vi "Utility Setup.vi"(8 "error in":errorcluster, 11 "VISA resource name":refnum<visa-resource-name>) -> (0 "error out":errorcluster, 3 "VISA resource name out":refnum<visa-resource-name>)   [LabVIEW 2011, in "GPT-9000.lvlib"]
uses:
  <instrlib>/GPT-9000/GPT-9000.lvlib
panel:
  in  "Setup Buzzer Sound for FAIL":T1={"Buzzer Sound"=0, "Duration Time(Sec)"=0.5} {"Duration Time(Sec)" min=0.2 max=999.9 step=0.1 format="%#.1f"; "Buzzer Sound" format="%b" items=["ON"=1, "OFF"=0]}
  in  "Setup Buzzer Sound for PASS":T1={"Buzzer Sound"=0, "Duration Time(Sec)"=0.5000000029802322} {"Duration Time(Sec)" min=0.20000000298023224 max=999.9000244140625 step=0.1 format="%#.1f"; "Buzzer Sound" format="%b" items=["ON"=1, "OFF"=0]}
  in  "Sets the brightness":u8(ring)=2 items=["bright"=2, "drak"=1]
  in  "Sets the contrast":u8(ring)=8 items=["8"=8, "7"=7, "6"=6, "5"=5, "4"=4, "3"=3, "2"=2, "1"=1]
  in  "SETUP":bool
  out "Query Buzzer Sound for FAIL":T2
  out "Query Buzzer Sound for PASS":T3
  out "Query the brightness":string
  out "Query the contrast":string
  out "ID Return String":string
  in  "Configure RS232 Baud Rate":u32(ring)=9600 items=["9600"=9600, "19200"=19200, "38400"=38400, "57600"=57600, "115200"=115200]
  in  "Clear Error(True)":bool=TRUE
  in  "ID Query (True)":bool=TRUE
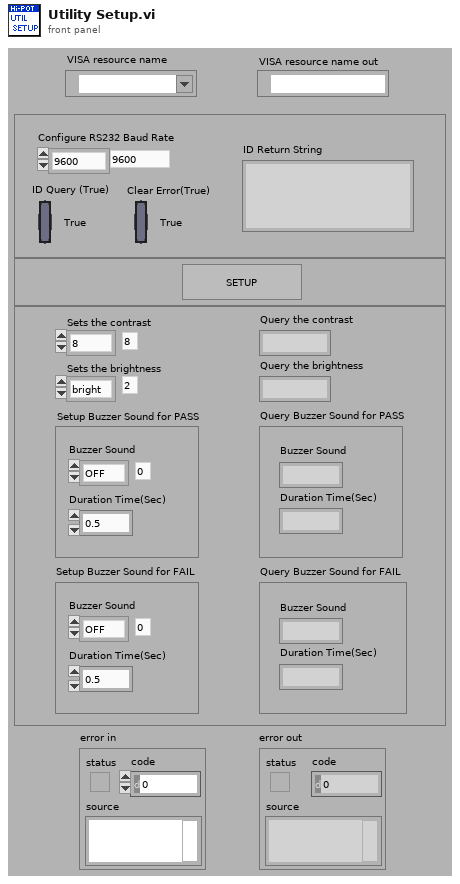
[diagram p1: front panel]
types:
  T1 = cluster{"Buzzer Sound":u8, "Duration Time(Sec)":dbl}
  T2 = cluster{"Duration Time(Sec)":string, "Buzzer Sound":string}
  T3 = cluster{"Buzzer Sound":string, "Duration Time(Sec)":string}
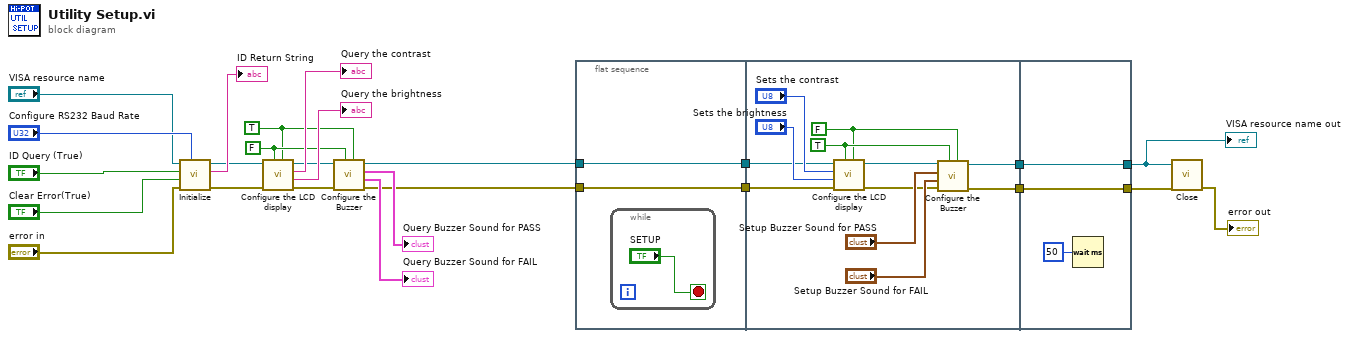
[diagram p0: block diagram]
diagram:
  w6 = TRUE ("Enable to Query")
  w7 = FALSE ("Enable to Setup")
  n1 = call <instrlib>:"Initialize.vi"("Configure RS232 Baud Rate"="Configure RS232 Baud Rate", "error in (no error)"="error in", "Clear Error(True)"="Clear Error(True)", "ID Query (True)"="ID Query (True)", "VISA resource name"="VISA resource name") -> ("error out"=w14:errorcluster, "ID Return String"=→"ID Return String":string, "VISA resource name out"=w15:refnum<visa-resource-name>)  [unwired: 3 in, 1 out]
  n2 = call <instrlib>:"Configure the LCD display.vi"("Enable to Query"=w6, "Enable to Setup"=w7, "error in"=w14, "VISA resource name"=w15) -> ("error out"=w12:errorcluster, "Query the brightness"=→"Query the brightness":string, "Query the contrast"=→"Query the contrast":string, "VISA resource name out"=w13:refnum<visa-resource-name>)  [unwired: 4 in]
  n3 = call <instrlib>:"Configure the Buzzer.vi"("Enable to Query"=w6, "Enable to Setup"=w7, "error in"=w12, "VISA resource name"=w13) -> ("error out"=w10:errorcluster, "Query Buzzer Sound for FAIL"=→"Query Buzzer Sound for FAIL":T2, "Query Buzzer Sound for PASS"=→"Query Buzzer Sound for PASS":T3, "VISA resource name out"=w11:refnum<visa-resource-name>)  [unwired: 4 in]
  n4 = flat-sequence {
    tunnel: w11 -> [w27]
    tunnel: w10 -> [w26]
    tunnel: [w27] -> w9
    tunnel: [w26] -> w8
    tunnel: w9 -> [w36]
    tunnel: w8 -> [w35]
    tunnel: [w32] -> w4
    tunnel: [w31] -> w3
    tunnel: [w42] -> w2
    tunnel: [w43] -> w1
    tunnel: w4 -> [w43]
    tunnel: w3 -> [w42]
    frame #0 {
      n5 = while {
        stop <- "SETUP" stop-if-true
      }
    }
    frame #1 {
      w29 = FALSE ("Enable to Query")
      w30 = TRUE ("Enable to Setup")
      n6 = call <instrlib>:"Configure the LCD display.vi"("Enable to Query"=w29, "Enable to Setup"=w30, "error in"=w35, "Sets the brightness"="Sets the brightness", "Sets the contrast"="Sets the contrast", "VISA resource name"=w36) -> ("error out"=w33:errorcluster, "VISA resource name out"=w34:refnum<visa-resource-name>)  [unwired: 2 in, 2 out]
      n7 = call <instrlib>:"Configure the Buzzer.vi"("Enable to Query"=w29, "Enable to Setup"=w30, "error in"=w33, "Setup Buzzer Sound for FAIL"="Setup Buzzer Sound for FAIL", "Setup Buzzer Sound for PASS"="Setup Buzzer Sound for PASS", "VISA resource name"=w34) -> ("error out"=w31:errorcluster, "VISA resource name out"=w32:refnum<visa-resource-name>)  [unwired: 2 in, 2 out]
    }
    frame #2 {
      n8 = Wait (ms)(milliseconds to wait=u32 50) -> ()  [unwired: 1 out]
    }
  }
  n9 = call <instrlib>:"Close.vi"("error in (no error)"=w2, "VISA resource name"=w1) -> ("error out"=→"error out":errorcluster)  [unwired: 9 in]
  "VISA resource name out" <- w1
